vi "status.vi"(7 "waitgroup":T1, 8 "error in (no error)":errorcluster) -> (0 "error out":errorcluster, 3 "active":i32)   [LabVIEW 2015, in "lv-waitgroup.lvlib"]
doc: "status.vi will take a given Waitgroup reference, pull the waitgroup ID and get the number of active processes."
uses:
  lv-waitgroup.lvlib
  _controls/api_waitgroup.ctl
  private/_controls/waitgroup.ctl
  _controls/data_error.ctl
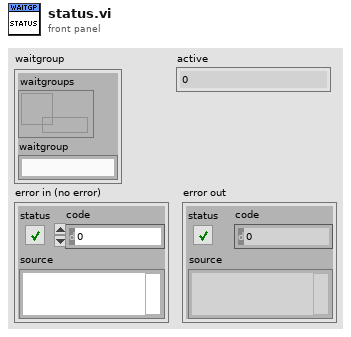
[diagram p1: front panel]
types:
  T1 = typedef "lv-waitgroup.lvlib/api_waitgroup.ctl" = cluster{"waitgroups":refnum<data-value>, "waitgroup":string}
  T2 = typedef "lv-waitgroup.lvlib/waitgroup.ctl" = cluster{"waitgroup":refnum<queue>, "queues":variant}
  T3 = typedef "lv-waitgroup.lvlib/data_error.ctl" = enum16{"<data_error>", "unable_to_generate_id", "waitgroup_not_found", "unable_to_add_to_waitgroup", "<null>"}
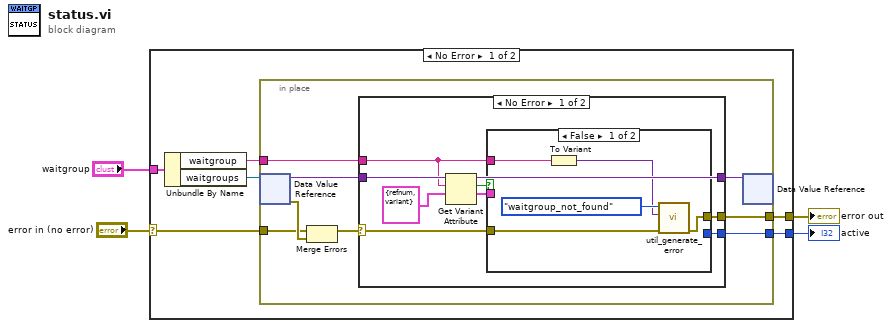
[diagram p0: block diagram]
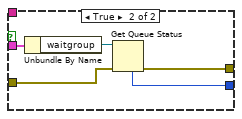
[diagram p2: hidden frame]
diagram:
  n1 = case shown="No Error" "error in (no error)" {
    selector: "error in (no error)" -> [w5 w40]
    tunnel: [w10 w40] -> w2
    tunnel: "waitgroup" -> [w8 _]
    tunnel: [w9 _] -> w1
    frame No Error {
      n2 = Unbundle By Name(w8) -> ("waitgroup"=w7:string, "waitgroups"=w6:refnum<data-value>)
      n3 = in-place {
        in-place-border: w5 -> [w17]
        in-place-border: [w15] -> w10
        in-place-border: [w14] -> w9
        in-place-border: w7 -> [w11]
        n4 = in-place-dvr #1(w6) -> (w16:variant, w18:errorcluster)
        n5 = Merge Errors(w17, w18) -> (w12:errorcluster)
        n6 = case shown="No Error" w12 {
          selector: w12 -> [w21 w38]
          tunnel: w16 -> [w25 w39]
          tunnel: [w24 w38] -> w15
          tunnel: [w23 _] -> w14
          tunnel: [w22 w39] -> w13
          tunnel: w11 -> [w19 _]
          frame No Error {
            n7 = Get Variant Attribute(Variant=w25, name=w19, default value (empty Variant)=T2 {"waitgroup"=refnum, "queues"=variant(refnum<queue>[] [])} ("shared_data")) -> (duplicate Variant=w22:variant, found=w20:bool, value=w26:T2)  [unwired: 1 in, 1 out]
            n8 = case shown="False" w20 {
              tunnel: w26 -> [_ w37]
              tunnel: [w30 w35] -> w24
              tunnel: [_ w34] -> w23
              tunnel: w21 -> [w31 w33]
              tunnel: w19 -> [w29 _]
              frame False {
                n9 = To Variant(anything=w29) -> (Variant=w28:variant)
                n10 = call "util_generate_error.vi"("error in (no error)"=w31, "data"=w28, "data_error"=data_error."waitgroup_not_found") -> ("error out"=w30:errorcluster)  [unwired: 8 in]
              }
              frame True {
                n11 = Unbundle By Name(w37) -> ("waitgroup"=w36:refnum<queue>)
                n12 = Get Queue Status(queue=w36, error in (no error)=w33) -> (error out=w35:errorcluster, # elements in queue=w34:i32)  [unwired: 1 in, 6 out]
              }
            }
          }
          frame Error {
          }
        }
        n13 = in-place-dvr #1(w13) -> ()  [unwired: 2 out]
      }
    }
    frame Error {
    }
  }
  "error out" <- w2
  "active" <- w1
